vi "simTC Global GUIDs.vi"() -> ()   [LabVIEW 2011, in "Simulated Thermocouple Custom Device.lvlib"]
uses:
  Simulated Thermocouple Custom Device.lvlib
panel:
  in  "Boolean":string="0461B564-03FA-16B1-4E9B-F524808B55DB"
  in  "TC Error":string="B4E1BD10-0157-C0E4-D269-AFE2C6056A58"
  in  "TC Calibration Config":string="3027efba-c0b5-45a3-8ca2-970824ba31f4"
  in  "TC Channel Config":string="b04bcaf6-e16e-4f2b-a421-09dcc5771ba7"
  in  "CO Channel Config":string="3b7fd3f7-897f-48c1-a62a-0ee2e9a994a1"
  in  "VO Channel Config":string="31dee1d3-8e49-4944-be8e-483cab571167"
  in  "Simulated Thermocouples":string="58e2782a-ff74-4e3c-99e5-d50d5b53a861"
  in  "Current Outputs":string="4997e311-51b7-4029-a044-e2490122e7ac"
  in  "Voltage Outputs":string="a01dde1d-2391-43a9-8263-697254600c9d"
  in  "Custom Device":string="32ef703f-981c-427b-acef-84d810e0c668"
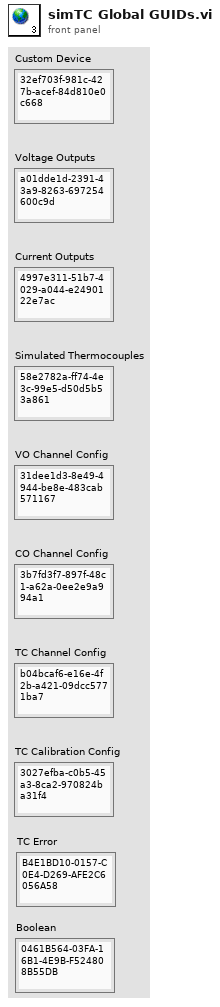
[diagram p1: front panel]
diagram:
